vi "FromRepo.vi"(8 "error in":errorcluster, 9 "from repo cluster":T2, 10 "repository in":refnum<class "NISE_CEF_Repository.lvclass">, 11 "node in":refnum<class "Page.lvclass">) -> (0 "error out":errorcluster, 2 "repository out":refnum<class "NISE_CEF_Repository.lvclass">, 3 "node":T1)   [LabVIEW 2015, in "Page.lvclass"]
doc: "Grabs information from the Repo and stores it in the nodes."
uses:
  Page.lvclass
  <vilib>/NI/Configuration Framework/Repository/NISE_CEF_Repository.lvclass
  <vilib>/NI/Configuration Framework/Node/FromRepoCluster.ctl
  <vilib>/NI/Configuration Framework/Node/NodeRef.ctl
  <vilib>/NI/Configuration Framework/Node/NISE_CEF_Node.lvclass
  CustomDeviceRepo/CustomDeviceRepo.lvclass
  Controls/RunTimeObjectTypes.ctl
  CustomDeviceRepo/CustomDeviceRepo.lvclass/CustomDeviceRepo.ctl
  Page.lvclass/Page.ctl
  CustomDeviceRepo/Read All Pages Properties.vi
  Write General Page Properties.vi
  Configuration Tool.lvlib
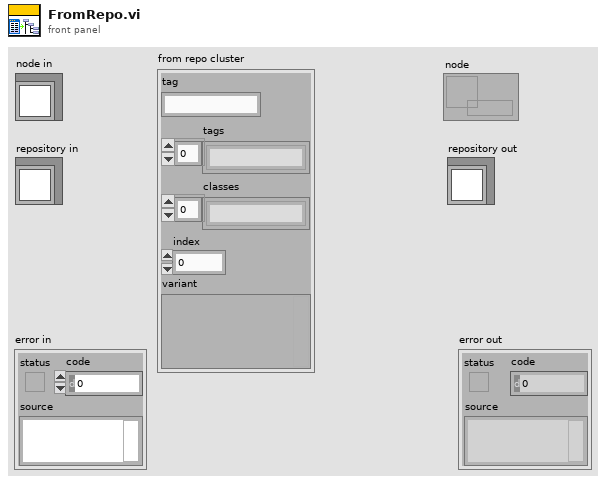
[diagram p1: front panel]
types:
  T1 = typedef "NISE_CEF_Node.lvclass/NodeRef.ctl" = refnum<data-value>
  T2 = typedef "NISE_CEF_Node.lvclass/FromRepoCluster.ctl" = cluster{"tag":string, "tags":string[], "classes":string[], "index":i32, "variant":variant}
  T3 = typedef "Configuration Tool.lvlib/RunTimeObjectTypes.ctl" = enum16{"ActionVIs", "ButtonList", "RunTimeMenu"}
  T4 = typedef "Page Properties.ctl" = cluster{"Name":string, "Disallow Renaming":bool, "Delete Protection":bool, "Exlcude from Alphabetical order":bool, "Allow Multi-Selection":bool, "GUID":string, "Parent GUIDs":string[], "Glyph":T5, "Inactive Glyph":T5, "Broken Glyph":T5, "Item to Launch":T5, "Additional Information":string, "Copy":enum16{"copy", "disabled"}, "Paste":enum16{"Create", "CreatIfNotExists_GUID", "CreatIfNotExists_Name", "Replace", "Dialog"}, "Help":T6}
  T5 = typedef "Path Cluster.ctl" = cluster{"Path":path, "Path Type":enum16{"Absolute", "To Base", "To Common Doc Dir", "To Application Data Dir"}}
  T6 = typedef "help.ctl" = cluster{"Item to Launch":T5, "Section":string, "File Type":enum16{"chm", "other"}}
  T7 = typedef "ActionVIs Properties.ctl" = cluster{"Action VI On Delete":T5, "Action VI On Load":T5, "Action VI On Paste":T5, "Action VI On Target Type Change":T5, "Action VI On Delete Request":T5, "Action VI On Compile":T5, "Action VI On System Shutdown":T5, "Action VI On Save":T5, "Action VI On Download":T5}
  T8 = typedef "ButtonLists Properties.ctl" = cluster{"ID":string, "Glyph":T5, "Button Type":T9, "Referenced GUID":string, "Button Text":string, "Caption":string, "Tip Strip":string, "Documentation":string, "Dependency":T10}
  T9 = typedef "Button Type.ctl" = enum16{"Action", "Dialog", "Page", "Notification", "Separator"}
  T10 = typedef "Dependency three item small.ctl" = cluster{"File Path Control":path, "Path Type":enum16{"Absolute", "To Base", "To Common Doc Dir", "To Application Data Dir"}, "Behavior":enum16{"Static", "Dynamic"}}
  T11 = typedef "RunTimeMenus Properties.ctl" = cluster{"GUID":string, "Execution":T12, "MinNrOfChilds":u32, "Name":string, "Item to Launch":T5, "Dependency":T10, "Custom Population":T5, "Menu Item Type":enum16{"Action", "VI", "Separator", "Custom"}, "Behavior":enum16{"Nothing", "Open Front Panel"}, "Position":enum16{"Centered", "Mouse Pointer"}}
  T12 = typedef "Execution Types.ctl" = enum16{"silent", "modal", "floating", "default"}
  T13 = cluster{"General Page Properties":T4, "ActionVIs Properties":T7, "Button List Properties":T8[], "RunTime Menus Properties":T11[]}[]
  T14 = cluster{"General Page Properties":T4, "ActionVIs Properties":T7, "Button List Properties":T8[], "RunTime Menus Properties":T11[]}
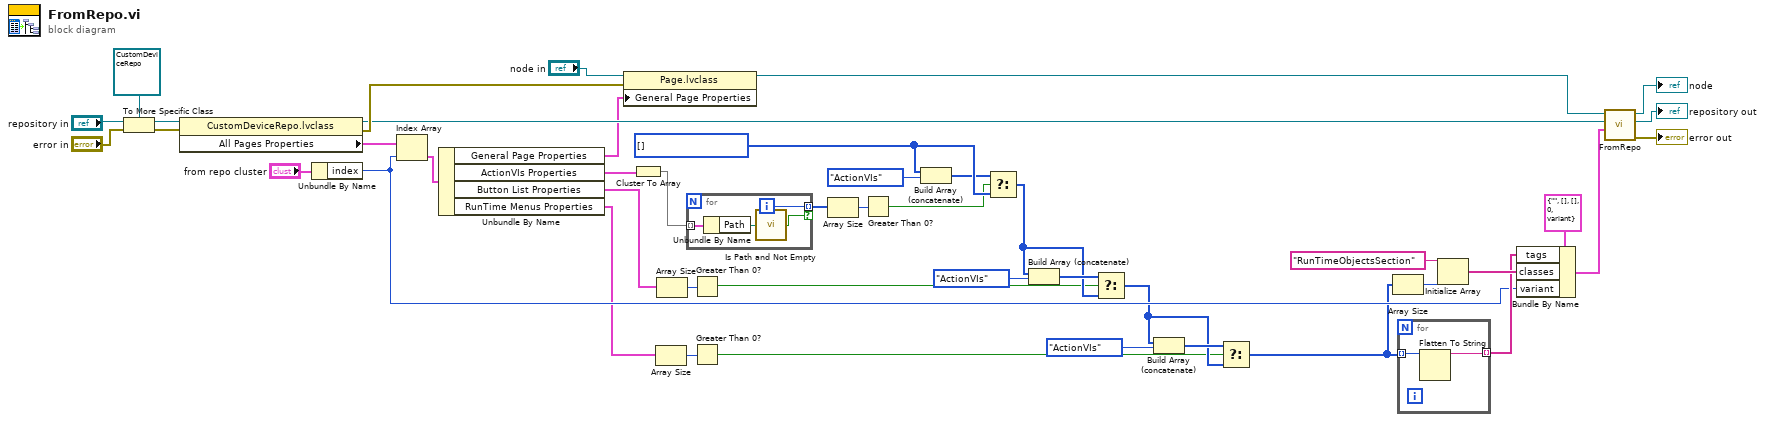
[diagram p0: block diagram]
diagram:
  w16 = T3[] [] items=["ActionVIs", "ButtonList", "RunTimeMenu"]
  n1 = To More Specific Class(target class=refnum<class "CustomDeviceRepo.lvclass"> refnum ("CustomDeviceRepo.lvclass"), reference="repository in", error in="error in") -> (specific class reference=w40:refnum<class "CustomDeviceRepo.lvclass">, error out=w39:errorcluster)
  n2 = property class="CustomDeviceRepo.lvclass"(reference=w40, error in=w39) -> (reference out=w32:refnum<class "CustomDeviceRepo.lvclass">, error out=w33:errorcluster, "All Pages Properties"=w35:T13)
  n3 = Unbundle By Name("from repo cluster") -> ("index"=w22:i32)
  n4 = Index Array(array=w35, index=w22) -> (element=w34:T14)
  n5 = Unbundle By Name(w34) -> ("General Page Properties"=w29:T4, "ActionVIs Properties"=w5:T7, "Button List Properties"=w20:T8[], "RunTime Menus Properties"=w21:T11[])
  n6 = property class="Page.lvclass"(reference="node in", error in=w33, "General Page Properties"=w29) -> (reference out=w31:refnum<class "Page.lvclass">)  [unwired: 1 out]
  n7 = Cluster To Array(cluster=w5) -> (array=w4:T5[])
  n8 = Array Size(array=w21) -> (size(s)=w18:i32)
  n9 = Array Size(array=w20) -> (size(s)=w19:i32)
  n10 = for {
    tunnel: [w48] -> w2 mode=indexing if=w45
    tunnel: w4 -> [w47] mode=indexing
    i -> [w48]
    n11 = Unbundle By Name(w47) -> ("Path"=w46:path)
    n12 = call <vilib>:"Is Path and Not Empty.vi"("path"=w46) -> ("Is Path and Not Empty?"=w45:bool)  [unwired: 4 in]
  }
  n13 = Greater Than 0?(x=w19) -> (x > 0?=w9:bool)
  n14 = Greater Than 0?(x=w18) -> (x > 0?=w7:bool)
  n15 = Array Size(array=w2) -> (size(s)=w3:i32)
  n16 = Greater Than 0?(x=w3) -> (x > 0?=w1:bool)
  n17 = Build Array (concatenate)(w16, RunTimeObjectTypes."ActionVIs" ("RunTimeObjectType")) -> (w15:T3[])
  n18 = Select(t=w15, s=w1, f=w16) -> (s? t:f=w10:T3[])
  n19 = Build Array (concatenate)(w10, RunTimeObjectTypes."ActionVIs" ("RunTimeObjectType")) -> (w14:T3[])
  n20 = Select(t=w14, s=w9, f=w10) -> (s? t:f=w8:T3[])
  n21 = Build Array (concatenate)(w8, RunTimeObjectTypes."ActionVIs" ("RunTimeObjectType")) -> (w11:T3[])
  n22 = Select(t=w11, s=w7, f=w8) -> (s? t:f=w6:T3[])
  n23 = Array Size(array=w6) -> (size(s)=w27:i32)
  n24 = for {
    tunnel: w6 -> [w50] mode=indexing
    tunnel: [w49] -> w24 mode=indexing
    n25 = Flatten To String(anything=w50) -> (data string=w49:string)  [unwired: 3 in, 2 out]
  }
  n26 = Initialize Array("RunTimeObjectsSection" ("element"), w27) -> (w25:string[])
  n27 = Bundle By Name(cluster=T2 {"tag"="", "tags"=[], "classes"=[], "index"=0, "variant"=variant} ("from repo cluster"), "tags"=w24, "classes"=w25, "variant"=w22) -> (w23:T2)
  n28 = call-parent "FromRepo.vi"("from repo cluster"=w23, "repository in"=w32, "node in"=w31) -> ("error out"=→"error out":errorcluster, "repository out"=→"repository out":refnum<class "NISE_CEF_Repository.lvclass">, "node"=→"node":T1)  [unwired: 6 in]
